vi "RangeCheck.vi"(0 "NhRegenGridSim in":refnum<class "NHRGridSim.lvclass">, 1 "RangeCheck":T1, 2 "Phase":i32, 3 "error in (no error)":errorcluster) -> (7 "NhRegenGridSim out":refnum<class "NHRGridSim.lvclass">, 10 "error out":errorcluster)   [LabVIEW 2018, in "AcPwrPlugins.lvlib" / "NHRGridSim.lvclass"]
doc: "This VI validates that the properties being set via the prefence dialog or stored in the INI file are valid."
uses:
  NHRGridSim.lvclass
  TypeDefs/RangeCheck.ctl
  <vilib>/Utility/error.llb/Error Cluster From Error Code.vi
  <vilib>/ErrorRing/Error Ring.xnode
  <instrlib>/NH Research 9400 Series/NH Research 9400 Series.lvlib
  <instrlib>/NH Research 9400 Series/Public/Utility/Query Capabilities (Frequency).vi
  <instrlib>/NH Research 9400 Series/Public/Utility/Query Capabilities (Power).vi
  <instrlib>/NH Research 9400 Series/Public/Utility/Query Capabilities (Current).vi
  <instrlib>/NH Research 9400 Series/Public/Utility/Query Capabilities (Voltage).vi
  <instrlib>/NH Research 9400 Series/Public/Utility/Query Capabilities (Phase Angle).vi
  <instrlib>/NH Research 9400 Series/Public/Utility/Query Capabilities (Sample).vi
  <instrlib>/NH Research 9400 Series/Public/Utility/Query Capabilities (Aperture).vi
  <instrlib>/NH Research 9400 Series/Public/Action-Status/Low Level/Query Range List (Voltage).vi
  <instrlib>/NH Research 9400 Series/Public/Action-Status/Low Level/Query Range List (Current).vi
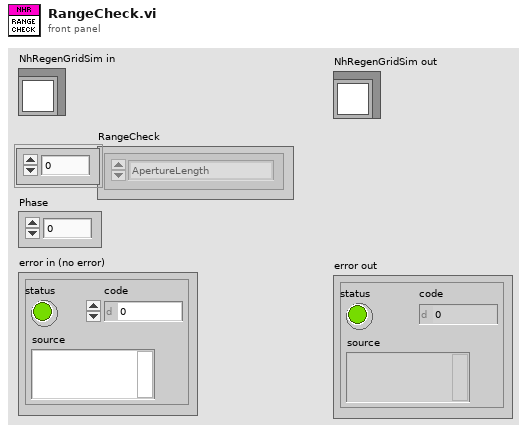
[diagram p1: front panel]
types:
  T1 = typedef "AcPwrPlugins.lvlib/NHRGridSim.lvclass/RangeCheck.ctl" = enum16{"ApertureLength", "NumberOfSamples", "SlewAngleMultiPhaseAB", "SlewAngleMultiPhaseAC", "RegulationGain", "VoltageRange", "CurrentRange", "PhaseAngle", "Power", "Current", "Voltage", "Frequency"}[]
  T2 = typedef "AcPwrPlugins.lvlib/NHRGridSim.lvclass/NHRGrid_Settings.ctl" = cluster{"MeasName":string, "Hardware":T3}
  T3 = typedef "AcPwrPlugins.lvlib/NHRGridSim.lvclass/NHRGrid_Hardware.ctl" = cluster{"Handle":string, "Reset":bool, "Mode":T4, "ID Query":bool, "Logical Instrument":T5}
  T4 = typedef "AcPwrPlugins.lvlib/NHRGridSim.lvclass/NHRGrid_Modes.ctl" = u8
  T5 = typedef "AcPwrPlugins.lvlib/NHRGridSim.lvclass/NHRGrid_Logical_Instrument.ctl" = cluster{"Name":string, "Vout (V)":dbl, "I limit (A)":dbl, "P limit (W)":dbl, "FreqOut (Hz)":dbl, "Ranges":cluster{"Voltage (V)":u16, "Current (A)":u16}, "Configure Instrument":u16, "Aperture (cycles)":i32, "AC Wave Shape":u16, "VType":string, "IType":string, "Phases":T6, "Slew Rates":T7, "Safety Trips":T8}[]
  T6 = typedef "AcPwrPlugins.lvlib/NHRGridSim.lvclass/NHRGrid_Phases.ctl" = cluster{"A-Volts (V)":dbl, "B-Volts (V)":dbl, "C-Volts (V)":dbl, "A-Curr (A)":dbl, "B-Curr (A)":dbl, "C-Curr (A)":dbl, "A-Power (W)":dbl, "B-Power (W)":dbl, "C-Power (W)":dbl, "Change at (Deg)":dbl, "B-Angle (Deg)":dbl, "C-Angle (Deg)":dbl}
  T7 = typedef "AcPwrPlugins.lvlib/NHRGridSim.lvclass/NHRGrid_SlewRates.ctl" = cluster{"Vmax (V/s)":dbl, "Vmin (V/s)":dbl, "Imax (A/s)":dbl, "Imin (A/s)":dbl, "Pmax (W/s)":dbl, "Pmin (W/s)":dbl, "Freq Max (Hz/s)":dbl, "Freq Min (Hz/s)":dbl, "Phase Angle Max (Deg/s)":dbl, "Phase Angle Min (Deg/s)":dbl}
  T8 = typedef "AcPwrPlugins.lvlib/NHRGridSim.lvclass/NHRGrid_SafetyTrips.ctl" = cluster{"Vmax (V)":dbl, "Vmin (V)":dbl, "Vmax Time (s)":dbl, "Vmin Time (s)":dbl, "Imax Source (A)":dbl, "Imax Sink (A)":dbl, "Imax Source Time (s)":dbl, "Imax Sink Time (s)":dbl, "Pmax Source (W)":dbl, "Pmax Sink (W)":dbl, "Pmax Source Time (s)":dbl, "Pmax Sink Time (s)":dbl, "Absolute Volt Peak":dbl, "Enable Volt Peak":bool, "Absolute Curr Peak":dbl, "Enable Curr Peak":bool}
  T9 = typedef "NH Research 9400 Series.lvlib/Range.ctl" = cluster{"Minimum":dbl, "Maximum":dbl}
  T10 = typedef "NH Research 9400 Series.lvlib/Current Capabilities.ctl" = cluster{"Module Min (A)":dbl, "Module Max (A)":dbl, "Range Min (A)":dbl, "Range Max (A)":dbl, "Measure Min (A)":dbl, "Measure Max (A)":dbl, "Measure Range Min (A)":dbl, "Measure Range Max (A)":dbl, "Slew Min (A per sec)":dbl, "Slew Max (A per sec)":dbl, "Slew Range Min (A per sec)":dbl, "Slew Range Max (A per sec)":dbl}
  T11 = typedef "NH Research 9400 Series.lvlib/Voltage Capabilities.ctl" = cluster{"Module Min (V)":dbl, "Module Max (V)":dbl, "Range Min (V)":dbl, "Range Max (V)":dbl, "Measure Min (V)":dbl, "Measure Max (V)":dbl, "Measure Range Min (V)":dbl, "Measure Range Max (V)":dbl, "Slew Min (V per sec)":dbl, "Slew Max (V per sec)":dbl, "Slew Range Min (V per sec)":dbl, "Slew Range Max (V per sec)":dbl}
  T12 = typedef "NH Research 9400 Series.lvlib/Power Capabilities.ctl" = cluster{"Module Min (W)":dbl, "Module Max (W)":dbl, "Range Min (W)":dbl, "Range Max (W)":dbl, "Slew Min (W per sec)":dbl, "Slew Max (W per sec)":dbl, "Slew Range Min (W per sec)":dbl, "Slew Range Max (W per sec)":dbl}
  T13 = typedef "NH Research 9400 Series.lvlib/Frequency Capabilities.ctl" = cluster{"Module Min (Hz)":dbl, "Module Max (Hz)":dbl, "Range Min (Hz)":dbl, "Range Max (Hz)":dbl, "Slew Min (Hz per sec)":dbl, "Slew Max (Hz per sec)":dbl, "Slew Range Min (Hz per sec)":dbl, "Slew Range Max (Hz per sec)":dbl}
  T14 = typedef "NH Research 9400 Series.lvlib/Phase Capabilities.ctl" = cluster{"Slew Min (deg per sec)":dbl, "Slew Max (deg per sec)":dbl, "Slew Range Min (deg per sec)":dbl, "Slew Range Max (deg per sec)":dbl}
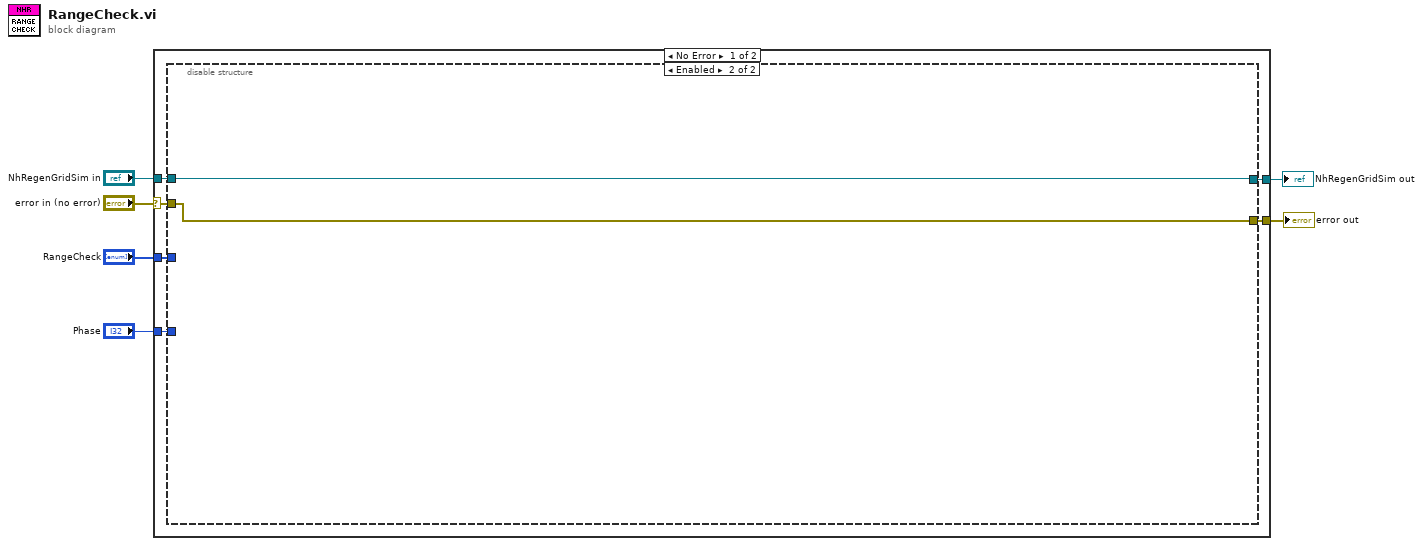
[diagram p0: block diagram]
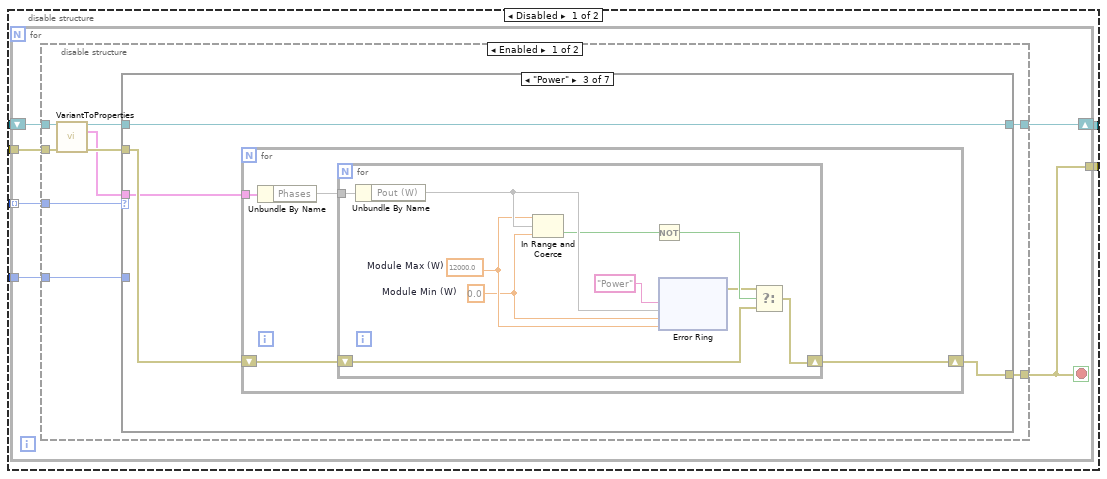
[diagram p2: hidden frame]
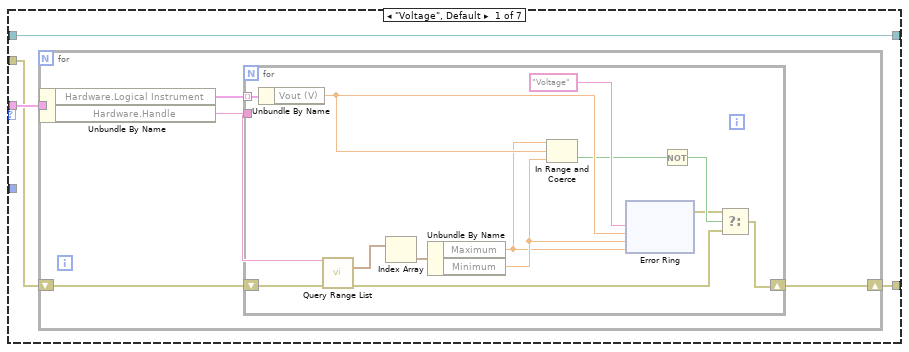
[diagram p3: hidden frame]
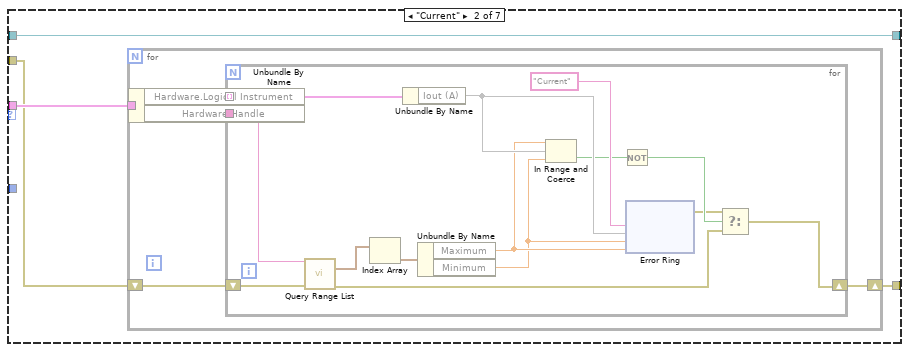
[diagram p4: hidden frame]
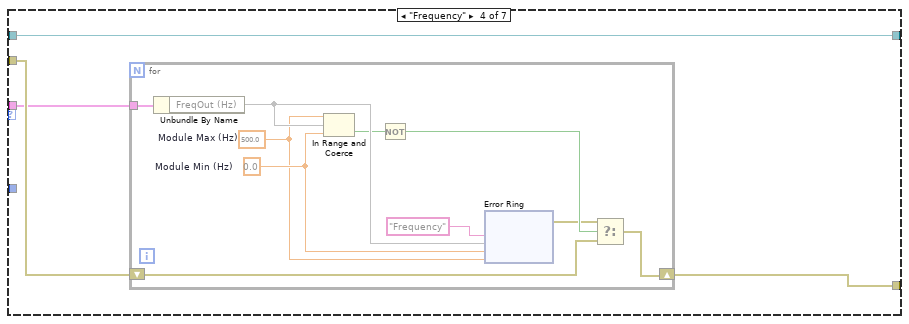
[diagram p5: hidden frame]
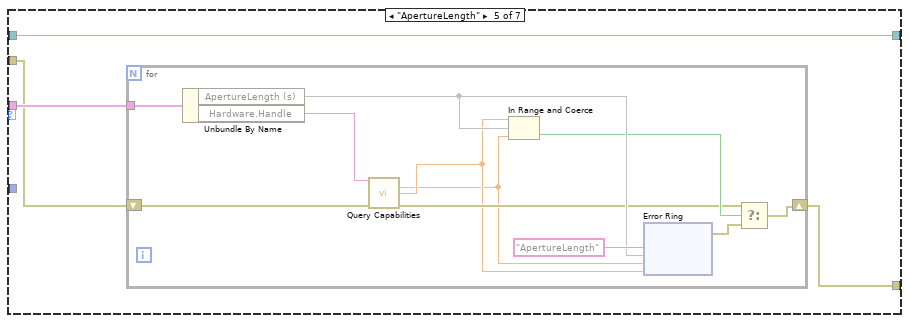
[diagram p6: hidden frame]
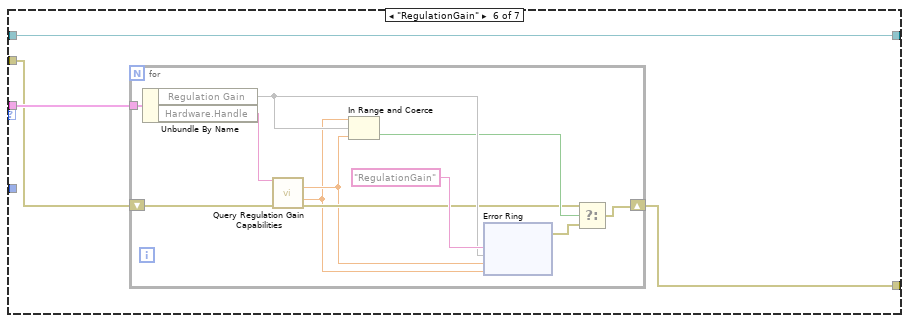
[diagram p7: hidden frame]
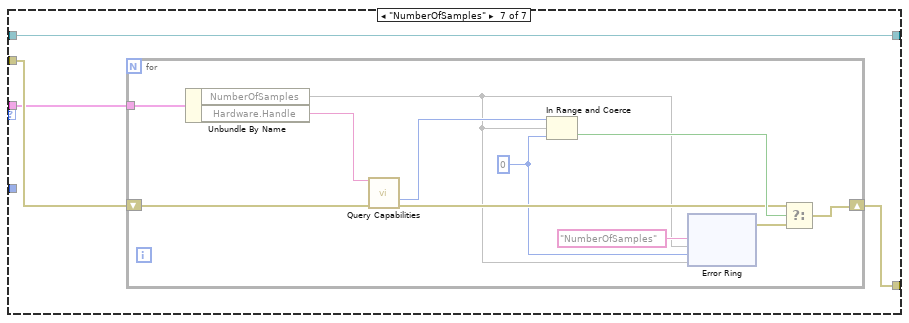
[diagram p8: hidden frame]
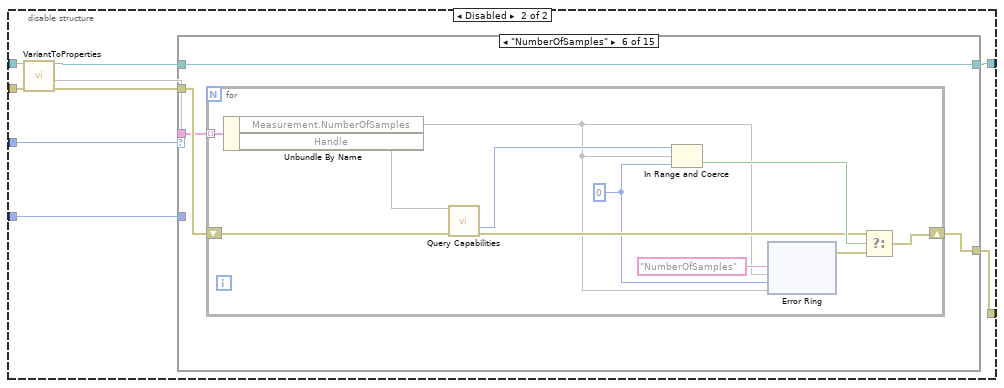
[diagram p9: hidden frame]
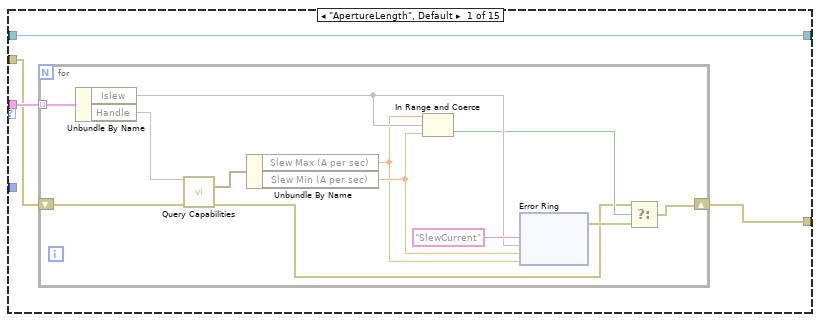
[diagram p10: hidden frame]
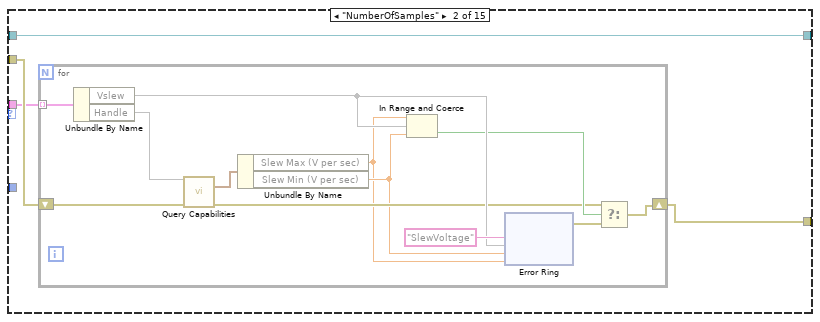
[diagram p11: hidden frame]
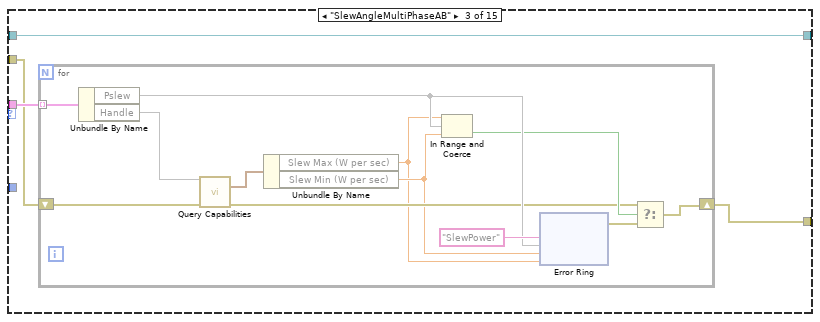
[diagram p12: hidden frame]
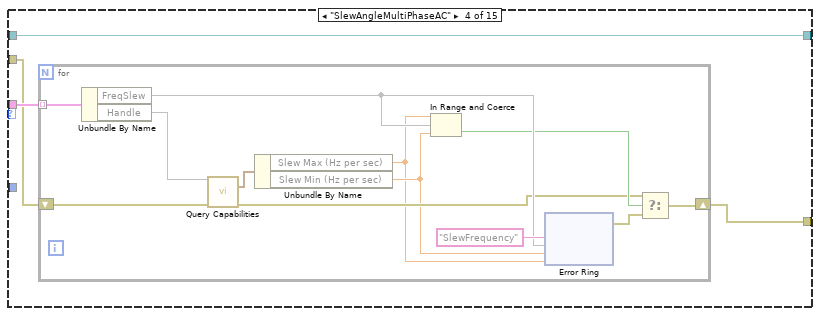
[diagram p13: hidden frame]
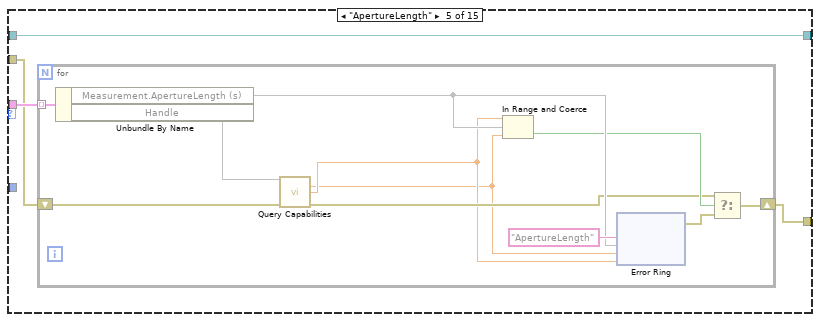
[diagram p14: hidden frame]
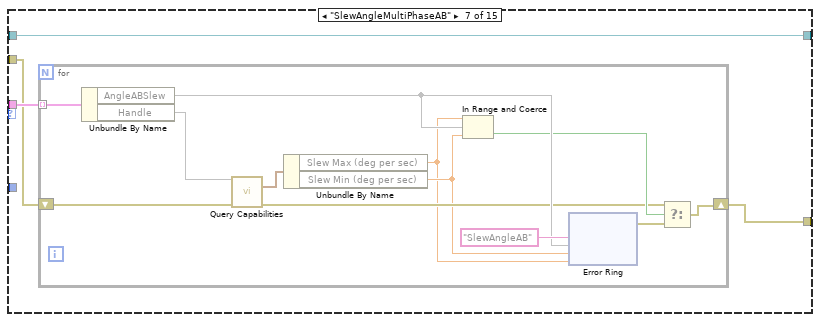
[diagram p15: hidden frame]
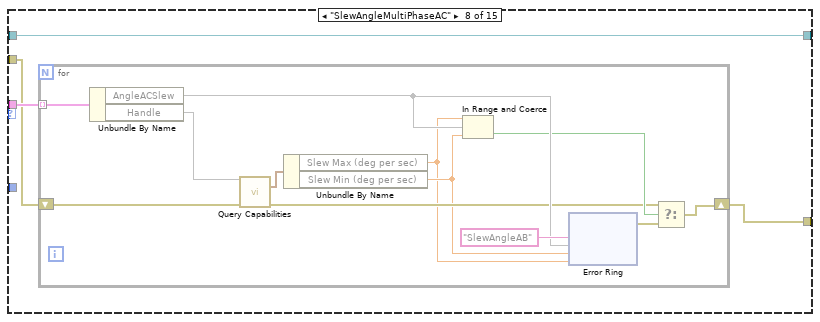
[diagram p16: hidden frame]
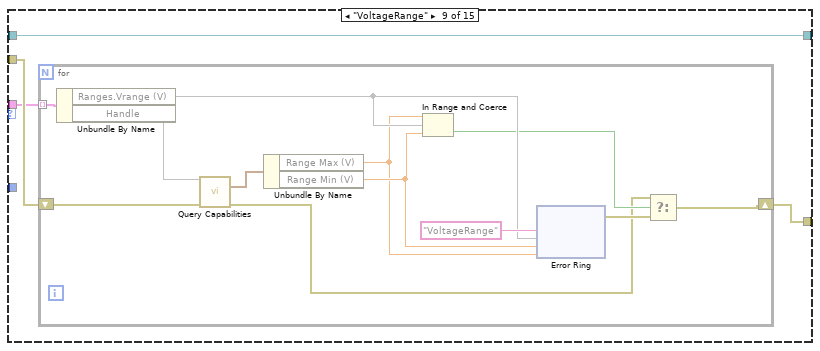
[diagram p17: hidden frame]
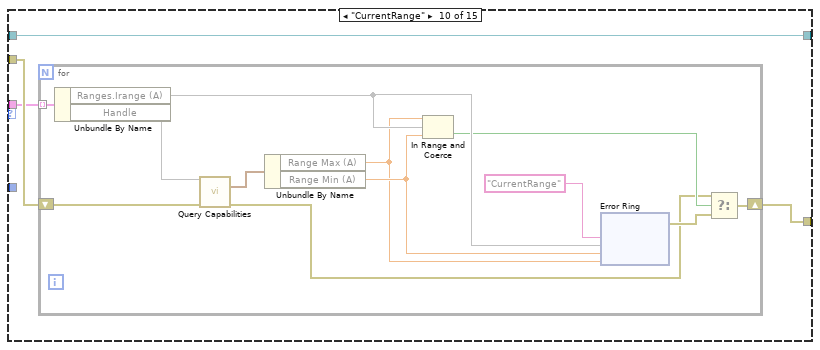
[diagram p18: hidden frame]
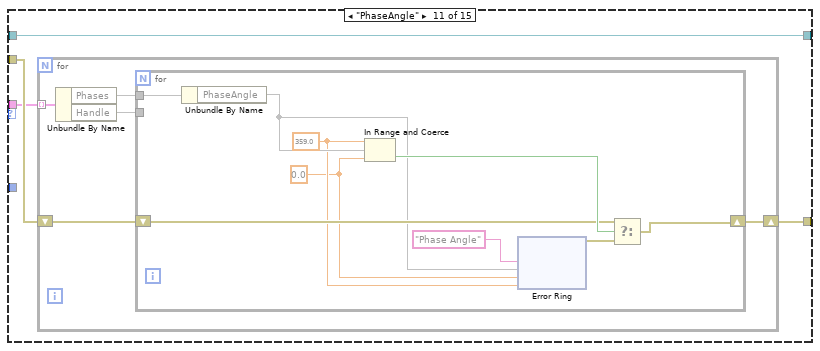
[diagram p19: hidden frame]
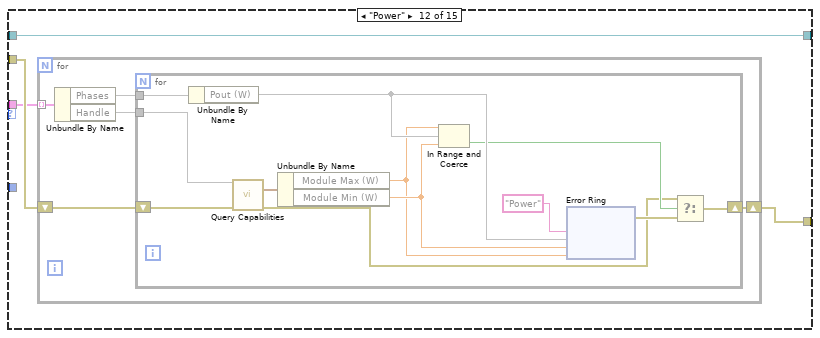
[diagram p20: hidden frame]
diagram:
  n1 = case shown="No Error" "error in (no error)" {
    selector: "error in (no error)" -> [w12 w641]
    tunnel: "Phase" -> [w11 _]
    tunnel: "NhRegenGridSim in" -> [w10 w642]
    tunnel: [w9 w642] -> w3
    tunnel: [w8 w641] -> w2
    tunnel: "RangeCheck" -> [w7 _]
    frame No Error {
      n2 = disable-structure shown="Enabled" {
        disable-tunnel: w12 -> [w18 w639]
        disable-tunnel: w11 -> [w17 _]
        disable-tunnel: w10 -> [w16 w640]
        disable-tunnel: [w15 w640] -> w9
        disable-tunnel: [w14 w639] -> w8
        disable-tunnel: w7 -> [w13 _]
        frame Disabled {
          n3 = for {
            tunnel: w13 -> [w24] mode=indexing
            tunnel: w17 -> [w23]
            shift-right: [w22] -> w15
            shift-left: w16 -> [w20]
            tunnel: [w21] -> w14
            tunnel: w18 -> [w19]
            stop <- w21 stop-if-true
            n4 = disable-structure shown="Enabled" {
              disable-tunnel: w24 -> [w33 w235]
              disable-tunnel: w23 -> [w32 w234]
              disable-tunnel: [w31 w233] -> w22
              disable-tunnel: [w30 w232] -> w21
              disable-tunnel: w20 -> [w29 w231]
              disable-tunnel: w19 -> [w28 w230]
              frame Enabled {
                n5 = call "VariantToProperties.vi"("NHRGridSim in"=w29, "error in (no error)"=w28) -> ("NHRGridSim out"=w26:refnum<class "NHRGridSim.lvclass">, "Device(s)Settings"=w25:T2, "error out"=w27:errorcluster)  [unwired: 8 in, 3 out]
                n6 = case shown="\"Power\"" w33 {
                  tunnel: w26 -> [w37 w70 w103 w130 w155 w180 w205]
                  tunnel: w32 -> [_ _ _ _ _ _ _]
                  tunnel: [w37 w70 w103 w130 w155 w180 w205] -> w31
                  tunnel: [w36 w69 w102 w131 w154 w179 w204] -> w30
                  tunnel: w27 -> [w34 w67 w101 w129 w152 w177 w203]
                  tunnel: w25 -> [w35 w68 w100 w128 w153 w178 w202]
                  frame "Voltage", Default {
                    n7 = for {
                      tunnel: w35 -> [w40]
                      shift-right: [w41] -> w36
                      shift-left: w34 -> [w42]
                      n8 = Unbundle By Name(w40) -> ("Hardware.Logical Instrument"=w39:T5, "Hardware.Handle"=w38:string)
                      n9 = for {
                        shift-right: [w55] -> w41
                        shift-left: w42 -> [w48]
                        tunnel: w39 -> [w54] mode=indexing
                        tunnel: w38 -> [w47]
                        n10 = Unbundle By Name(w54) -> ("Vout (V)"=w53:dbl)
                        n11 = call-poly <instrlib>:"Query Range List.vi"("VISA resource name"=w47, "error in (no error)"=w48) -> ("Voltage Range List (V)"=w46:T9[], "error out"=w49:errorcluster)  [unwired: 11 in, 1 out]
                        n12 = Index Array(array=w46) -> (element=w45:T9)  [unwired: 1 in]
                        n13 = Unbundle By Name(w45) -> ("Maximum"=w43:dbl, "Minimum"=w44:dbl)
                        n14 = In Range and Coerce(upper limit=w43, x=w53, lower limit=w44) -> (In Range?=w52:bool)  [unwired: 1 out]
                        n15 = xnode "Error Ring"("parameter 0"="Voltage", "parameter 1"=w53, "parameter 2"=w44, "parameter 3"=w43) -> ("error out"=w50:errorcluster)
                        n16 = Not(x=w52) -> (.not. x?=w51:bool)
                        n17 = Select(t=w50, s=w51, f=w49) -> (s? t:f=w55:errorcluster)
                      }
                    }
                  }
                  frame "Current" {
                    n18 = for {
                      tunnel: w68 -> [w73]
                      shift-right: [w74] -> w69
                      shift-left: w67 -> [w75]
                      n19 = Unbundle By Name(w73) -> ("Hardware.Logical Instrument"=w72:T5, "Hardware.Handle"=w71:string)
                      n20 = for {
                        shift-right: [w88] -> w74
                        shift-left: w75 -> [w81]
                        tunnel: w72 -> [w87] mode=indexing
                        tunnel: w71 -> [w79]
                        n21 = call-poly <instrlib>:"Query Range List.vi"("VISA resource name"=w79, "error in (no error)"=w81) -> ("Current Range List (A)"=w82:T9[], "error out"=w80:errorcluster)  [unwired: 11 in, 1 out]
                        n22 = Index Array(array=w82) -> (element=w78:T9)  [unwired: 1 in]
                        n23 = Unbundle By Name(w87) -> ("Iout (A)"=w86)
                        n24 = Unbundle By Name(w78) -> ("Maximum"=w77:dbl, "Minimum"=w76:dbl)
                        n25 = In Range and Coerce(upper limit=w77, x=w86, lower limit=w76) -> (In Range?=w85:bool)  [unwired: 1 out]
                        n26 = Not(x=w85) -> (.not. x?=w84:bool)
                        n27 = xnode "Error Ring"("parameter 0"="Current", "parameter 1"=w86, "parameter 2"=w76, "parameter 3"=w77) -> ("error out"=w83:errorcluster)
                        n28 = Select(t=w83, s=w84, f=w80) -> (s? t:f=w88:errorcluster)
                      }
                    }
                  }
                  frame "Power" {
                    n29 = for {
                      tunnel: w100 -> [w105]
                      shift-right: [w106] -> w102
                      shift-left: w101 -> [w107]
                      n30 = Unbundle By Name(w105) -> ("Phases"=w104)
                      n31 = for {
                        shift-right: [w116] -> w106
                        shift-left: w107 -> [w109]
                        tunnel: w104 -> [w115]
                        w112 = 0.0  # Module Min (W)
                        w113 = 12000.0  # Module Max (W)
                        n32 = Unbundle By Name(w115) -> ("Pout (W)"=w114)
                        n33 = In Range and Coerce(upper limit=w113, x=w114, lower limit=w112) -> (In Range?=w111:bool)  [unwired: 1 out]
                        n34 = Not(x=w111) -> (.not. x?=w110:bool)
                        n35 = xnode "Error Ring"("parameter 0"="Power", "parameter 1"=w114, "parameter 2"=w112, "parameter 3"=w113) -> ("error out"=w108:errorcluster)
                        n36 = Select(t=w108, s=w110, f=w109) -> (s? t:f=w116:errorcluster)
                      }
                    }
                  }
                  frame "Frequency" {
                    n37 = for {
                      tunnel: w128 -> [w139]
                      shift-right: [w140] -> w131
                      shift-left: w129 -> [w138]
                      w133 = 0.0  # Module Min (Hz)
                      w132 = 500.0  # Module Max (Hz)
                      n38 = Unbundle By Name(w139) -> ("FreqOut (Hz)"=w137)
                      n39 = In Range and Coerce(upper limit=w132, x=w137, lower limit=w133) -> (In Range?=w136:bool)  [unwired: 1 out]
                      n40 = Not(x=w136) -> (.not. x?=w135:bool)
                      n41 = xnode "Error Ring"("parameter 0"="Frequency", "parameter 1"=w137, "parameter 2"=w133, "parameter 3"=w132) -> ("error out"=w134:errorcluster)
                      n42 = Select(t=w134, s=w135, f=w138) -> (s? t:f=w140:errorcluster)
                    }
                  }
                  frame "ApertureLength" {
                    n43 = for {
                      tunnel: w153 -> [w163]
                      shift-right: [w164] -> w154
                      shift-left: w152 -> [w161]
                      n44 = Unbundle By Name(w163) -> ("ApertureLength (s)"=w160, "Hardware.Handle"=w162:string)
                      n45 = call-poly <instrlib>:"Query Capabilities.vi"("VISA resource name"=w162, "error in (no error)"=w161) -> ("Aperture Min (s)"=w156:dbl, "Aperture Max (s)"=w157:dbl, "error out"=w158:errorcluster)  [unwired: 10 in, 1 out]
                      n46 = In Range and Coerce(upper limit=w157, x=w160, lower limit=w156) -> (In Range?=w159:bool)  [unwired: 1 out]
                      n47 = xnode "Error Ring"("parameter 0"="ApertureLength", "parameter 1"=w160, "parameter 2"=w156, "parameter 3"=w157) -> ("error out"=w165:errorcluster)
                      n48 = Select(t=w158, s=w159, f=w165) -> (s? t:f=w164:errorcluster)
                    }
                  }
                  frame "RegulationGain" {
                    n49 = for {
                      tunnel: w178 -> [w188]
                      shift-right: [w189] -> w179
                      shift-left: w177 -> [w186]
                      n50 = Unbundle By Name(w188) -> ("Regulation Gain"=w185, "Hardware.Handle"=w187:string)
                      n51 = call <instrlib>:"Query Regulation Gain Capabilities.vi"("VISA resource name"=w187, "error in (no error)"=w186) -> ("Minimum"=w182:dbl, "Maximum"=w181:dbl, "error out"=w183:errorcluster)  [unwired: 9 in, 2 out]
                      n52 = In Range and Coerce(upper limit=w181, x=w185, lower limit=w182) -> (In Range?=w184:bool)  [unwired: 1 out]
                      n53 = xnode "Error Ring"("parameter 0"="RegulationGain", "parameter 1"=w185, "parameter 2"=w182, "parameter 3"=w181) -> ("error out"=w190:errorcluster)
                      n54 = Select(t=w183, s=w184, f=w190) -> (s? t:f=w189:errorcluster)
                    }
                  }
                  frame "NumberOfSamples" {
                    n55 = for {
                      tunnel: w202 -> [w213]
                      shift-right: [w214] -> w204
                      shift-left: w203 -> [w211]
                      w207 = u32 0 ("lower limit")
                      n56 = Unbundle By Name(w213) -> ("NumberOfSamples"=w206, "Hardware.Handle"=w212:string)
                      n57 = call-poly <instrlib>:"Query Capabilities.vi"("VISA resource name"=w212, "error in (no error)"=w211) -> ("Points"=w208:u32, "error out"=w209:errorcluster)  [unwired: 9 in, 3 out]
                      n58 = In Range and Coerce(upper limit=w208, x=w206, lower limit=w207) -> (In Range?=w210:bool)  [unwired: 1 out]
                      n59 = xnode "Error Ring"("parameter 0"="NumberOfSamples", "parameter 1"=w206, "parameter 2"=w207, "parameter 3"=w206) -> ("error out"=w215:errorcluster)
                      n60 = Select(t=w209, s=w210, f=w215) -> (s? t:f=w214:errorcluster)
                    }
                  }
                }
              }
              frame Disabled {
                n61 = call "VariantToProperties.vi"("NHRGridSim in"=w231, "error in (no error)"=w230) -> ("NHRGridSim out"=w228:refnum<class "NHRGridSim.lvclass">, 14:w227, "error out"=w229:errorcluster)  [unwired: 7 in, 4 out]
                n62 = case shown="\"NumberOfSamples\"" w235 {
                  tunnel: w228 -> [w239 w265 w291 w317 w343 w368 w393 w419 w445 w471 w497 w525 w556 w585 w615]
                  tunnel: w234 -> [_ _ _ _ _ _ _ _ _ _ _ _ _ _ _]
                  tunnel: [w239 w265 w291 w317 w343 w368 w393 w419 w445 w471 w497 w525 w556 w585 w615] -> w233
                  tunnel: [w238 w264 w290 w316 w342 w367 w392 w418 w444 w470 w496 w524 w555 w584 w616] -> w232
                  tunnel: w229 -> [w236 w263 w288 w314 w340 w366 w390 w416 w443 w469 w495 w523 w554 w582 w614]
                  tunnel: w227 -> [w237 w262 w289 w315 w341 w365 w391 w417 w442 w468 w494 w522 w553 w583 w613]
                  frame "ApertureLength", Default {
                    n63 = for {
                      tunnel: w237 -> [w248] mode=indexing
                      shift-right: [w249] -> w238
                      shift-left: w236 -> [w246]
                      n64 = Unbundle By Name(w248) -> ("Islew"=w244, "Handle"=w247)
                      n65 = call-poly <instrlib>:"Query Capabilities.vi"("VISA resource name"=w247, "error in (no error)"=w246) -> ("Current Capabilities"=w245:T10, "error out"=w240:errorcluster)  [unwired: 11 in, 1 out]
                      n66 = Unbundle By Name(w245) -> ("Slew Max (A per sec)"=w241:dbl, "Slew Min (A per sec)"=w242:dbl)
                      n67 = In Range and Coerce(upper limit=w241, x=w244, lower limit=w242) -> (In Range?=w243:bool)  [unwired: 1 out]
                      n68 = xnode "Error Ring"("parameter 0"="SlewCurrent", "parameter 1"=w244, "parameter 2"=w242, "parameter 3"=w241) -> ("error out"=w250:errorcluster)
                      n69 = Select(t=w240, s=w243, f=w250) -> (s? t:f=w249:errorcluster)
                    }
                  }
                  frame "NumberOfSamples" {
                    n70 = for {
                      tunnel: w262 -> [w274] mode=indexing
                      shift-right: [w275] -> w264
                      shift-left: w263 -> [w272]
                      n71 = Unbundle By Name(w274) -> ("Vslew"=w270, "Handle"=w273)
                      n72 = call-poly <instrlib>:"Query Capabilities.vi"("VISA resource name"=w273, "error in (no error)"=w272) -> ("Voltage Capabilities"=w271:T11, "error out"=w268:errorcluster)  [unwired: 11 in, 1 out]
                      n73 = Unbundle By Name(w271) -> ("Slew Max (V per sec)"=w266:dbl, "Slew Min (V per sec)"=w267:dbl)
                      n74 = In Range and Coerce(upper limit=w266, x=w270, lower limit=w267) -> (In Range?=w269:bool)  [unwired: 1 out]
                      n75 = xnode "Error Ring"("parameter 0"="SlewVoltage", "parameter 1"=w270, "parameter 2"=w267, "parameter 3"=w266) -> ("error out"=w276:errorcluster)
                      n76 = Select(t=w268, s=w269, f=w276) -> (s? t:f=w275:errorcluster)
                    }
                  }
                  frame "SlewAngleMultiPhaseAB" {
                    n77 = for {
                      tunnel: w289 -> [w300] mode=indexing
                      shift-right: [w301] -> w290
                      shift-left: w288 -> [w298]
                      n78 = Unbundle By Name(w300) -> ("Pslew"=w296, "Handle"=w299)
                      n79 = call-poly <instrlib>:"Query Capabilities.vi"("VISA resource name"=w299, "error in (no error)"=w298) -> ("Power Capabilities"=w297:T12, "error out"=w294:errorcluster)  [unwired: 11 in, 1 out]
                      n80 = Unbundle By Name(w297) -> ("Slew Max (W per sec)"=w292:dbl, "Slew Min (W per sec)"=w293:dbl)
                      n81 = In Range and Coerce(upper limit=w292, x=w296, lower limit=w293) -> (In Range?=w295:bool)  [unwired: 1 out]
                      n82 = xnode "Error Ring"("parameter 0"="SlewPower", "parameter 1"=w296, "parameter 2"=w293, "parameter 3"=w292) -> ("error out"=w302:errorcluster)
                      n83 = Select(t=w294, s=w295, f=w302) -> (s? t:f=w301:errorcluster)
                    }
                  }
                  frame "SlewAngleMultiPhaseAC" {
                    n84 = for {
                      tunnel: w315 -> [w326] mode=indexing
                      shift-right: [w327] -> w316
                      shift-left: w314 -> [w324]
                      n85 = Unbundle By Name(w326) -> ("FreqSlew"=w322, "Handle"=w325)
                      n86 = call-poly <instrlib>:"Query Capabilities.vi"("VISA resource name"=w325, "error in (no error)"=w324) -> ("Frequency Capabilities"=w323:T13, "error out"=w320:errorcluster)  [unwired: 11 in, 1 out]
                      n87 = Unbundle By Name(w323) -> ("Slew Max (Hz per sec)"=w318:dbl, "Slew Min (Hz per sec)"=w319:dbl)
                      n88 = In Range and Coerce(upper limit=w318, x=w322, lower limit=w319) -> (In Range?=w321:bool)  [unwired: 1 out]
                      n89 = xnode "Error Ring"("parameter 0"="SlewFrequency", "parameter 1"=w322, "parameter 2"=w319, "parameter 3"=w318) -> ("error out"=w328:errorcluster)
                      n90 = Select(t=w320, s=w321, f=w328) -> (s? t:f=w327:errorcluster)
                    }
                  }
                  frame "ApertureLength" {
                    n91 = for {
                      tunnel: w341 -> [w351] mode=indexing
                      shift-right: [w352] -> w342
                      shift-left: w340 -> [w349]
                      n92 = Unbundle By Name(w351) -> ("Measurement.ApertureLength (s)"=w348, "Handle"=w350)
                      n93 = call-poly <instrlib>:"Query Capabilities.vi"("VISA resource name"=w350, "error in (no error)"=w349) -> ("Aperture Min (s)"=w344:dbl, "Aperture Max (s)"=w345:dbl, "error out"=w346:errorcluster)  [unwired: 10 in, 1 out]
                      n94 = In Range and Coerce(upper limit=w345, x=w348, lower limit=w344) -> (In Range?=w347:bool)  [unwired: 1 out]
                      n95 = xnode "Error Ring"("parameter 0"="ApertureLength", "parameter 1"=w348, "parameter 2"=w344, "parameter 3"=w345) -> ("error out"=w353:errorcluster)
                      n96 = Select(t=w346, s=w347, f=w353) -> (s? t:f=w352:errorcluster)
                    }
                  }
                  frame "NumberOfSamples" {
                    n97 = for {
                      tunnel: w365 -> [w376] mode=indexing
                      shift-right: [w377] -> w367
                      shift-left: w366 -> [w374]
                      w370 = u32 0 ("lower limit")
                      n98 = Unbundle By Name(w376) -> ("Measurement.NumberOfSamples"=w369, "Handle"=w375)
                      n99 = call-poly <instrlib>:"Query Capabilities.vi"("VISA resource name"=w375, "error in (no error)"=w374) -> ("Points"=w371:u32, "error out"=w372:errorcluster)  [unwired: 9 in, 3 out]
                      n100 = In Range and Coerce(upper limit=w371, x=w369, lower limit=w370) -> (In Range?=w373:bool)  [unwired: 1 out]
                      n101 = xnode "Error Ring"("parameter 0"="NumberOfSamples", "parameter 1"=w369, "parameter 2"=w370, "parameter 3"=w369) -> ("error out"=w378:errorcluster)
                      n102 = Select(t=w372, s=w373, f=w378) -> (s? t:f=w377:errorcluster)
                    }
                  }
                  frame "SlewAngleMultiPhaseAB" {
                    n103 = for {
                      tunnel: w391 -> [w402] mode=indexing
                      shift-right: [w403] -> w392
                      shift-left: w390 -> [w400]
                      n104 = Unbundle By Name(w402) -> ("AngleABSlew"=w398, "Handle"=w401)
                      n105 = call-poly <instrlib>:"Query Capabilities.vi"("VISA resource name"=w401, "error in (no error)"=w400) -> ("Phase Angle Capabilities"=w399:T14, "error out"=w396:errorcluster)  [unwired: 11 in, 1 out]
                      n106 = Unbundle By Name(w399) -> ("Slew Max (deg per sec)"=w394:dbl, "Slew Min (deg per sec)"=w395:dbl)
                      n107 = In Range and Coerce(upper limit=w394, x=w398, lower limit=w395) -> (In Range?=w397:bool)  [unwired: 1 out]
                      n108 = xnode "Error Ring"("parameter 0"="SlewAngleAB", "parameter 1"=w398, "parameter 2"=w395, "parameter 3"=w394) -> ("error out"=w404:errorcluster)
                      n109 = Select(t=w396, s=w397, f=w404) -> (s? t:f=w403:errorcluster)
                    }
                  }
                  frame "SlewAngleMultiPhaseAC" {
                    n110 = for {
                      tunnel: w417 -> [w428] mode=indexing
                      shift-right: [w429] -> w418
                      shift-left: w416 -> [w426]
                      n111 = Unbundle By Name(w428) -> ("AngleACSlew"=w424, "Handle"=w427)
                      n112 = call-poly <instrlib>:"Query Capabilities.vi"("VISA resource name"=w427, "error in (no error)"=w426) -> ("Phase Angle Capabilities"=w425:T14, "error out"=w422:errorcluster)  [unwired: 11 in, 1 out]
                      n113 = Unbundle By Name(w425) -> ("Slew Max (deg per sec)"=w420:dbl, "Slew Min (deg per sec)"=w421:dbl)
                      n114 = In Range and Coerce(upper limit=w420, x=w424, lower limit=w421) -> (In Range?=w423:bool)  [unwired: 1 out]
                      n115 = xnode "Error Ring"("parameter 0"="SlewAngleAB", "parameter 1"=w424, "parameter 2"=w421, "parameter 3"=w420) -> ("error out"=w430:errorcluster)
                      n116 = Select(t=w422, s=w423, f=w430) -> (s? t:f=w429:errorcluster)
                    }
                  }
                  frame "VoltageRange" {
                    n117 = for {
                      tunnel: w442 -> [w454] mode=indexing
                      shift-right: [w455] -> w444
                      shift-left: w443 -> [w452]
                      n118 = Unbundle By Name(w454) -> ("Ranges.Vrange (V)"=w450, "Handle"=w453)
                      n119 = call-poly <instrlib>:"Query Capabilities.vi"("VISA resource name"=w453, "error in (no error)"=w452) -> ("Voltage Capabilities"=w451:T11, "error out"=w446:errorcluster)  [unwired: 11 in, 1 out]
                      n120 = Unbundle By Name(w451) -> ("Range Max (V)"=w447:dbl, "Range Min (V)"=w448:dbl)
                      n121 = In Range and Coerce(upper limit=w447, x=w450, lower limit=w448) -> (In Range?=w449:bool)  [unwired: 1 out]
                      n122 = xnode "Error Ring"("parameter 0"="VoltageRange", "parameter 1"=w450, "parameter 2"=w448, "parameter 3"=w447) -> ("error out"=w456:errorcluster)
                      n123 = Select(t=w446, s=w449, f=w456) -> (s? t:f=w455:errorcluster)
                    }
                  }
                  frame "CurrentRange" {
                    n124 = for {
                      tunnel: w468 -> [w480] mode=indexing
                      shift-right: [w481] -> w470
                      shift-left: w469 -> [w478]
                      n125 = Unbundle By Name(w480) -> ("Ranges.Irange (A)"=w476, "Handle"=w479)
                      n126 = call-poly <instrlib>:"Query Capabilities.vi"("VISA resource name"=w479, "error in (no error)"=w478) -> ("Current Capabilities"=w477:T10, "error out"=w472:errorcluster)  [unwired: 11 in, 1 out]
                      n127 = Unbundle By Name(w477) -> ("Range Max (A)"=w473:dbl, "Range Min (A)"=w474:dbl)
                      n128 = In Range and Coerce(upper limit=w473, x=w476, lower limit=w474) -> (In Range?=w475:bool)  [unwired: 1 out]
                      n129 = xnode "Error Ring"("parameter 0"="CurrentRange", "parameter 1"=w476, "parameter 2"=w474, "parameter 3"=w473) -> ("error out"=w482:errorcluster)
                      n130 = Select(t=w472, s=w475, f=w482) -> (s? t:f=w481:errorcluster)
                    }
                  }
                  frame "PhaseAngle" {
                    n131 = for {
                      tunnel: w494 -> [w500] mode=indexing
                      shift-right: [w501] -> w496
                      shift-left: w495 -> [w502]
                      n132 = Unbundle By Name(w500) -> ("Phases"=w499, "Handle"=w498)
                      n133 = for {
                        shift-right: [w509] -> w501
                        shift-left: w502 -> [w506]
                        tunnel: w499 -> [w508]
                        tunnel: w498 -> [_]
                        w504 = 359.0 ("Slew Max (deg per sec)")
                        w503 = 0.0 ("Slew Max (deg per sec)")
                        n134 = Unbundle By Name(w508) -> ("PhaseAngle"=w505)
                        n135 = In Range and Coerce(upper limit=w504, x=w505, lower limit=w503) -> (In Range?=w507:bool)  [unwired: 1 out]
                        n136 = xnode "Error Ring"("parameter 0"="Phase Angle", "parameter 1"=w505, "parameter 2"=w503, "parameter 3"=w504) -> ("error out"=w510:errorcluster)
                        n137 = Select(t=w506, s=w507, f=w510) -> (s? t:f=w509:errorcluster)
                      }
                    }
                  }
                  frame "Power" {
                    n138 = for {
                      tunnel: w522 -> [w528] mode=indexing
                      shift-right: [w529] -> w524
                      shift-left: w523 -> [w530]
                      n139 = Unbundle By Name(w528) -> ("Phases"=w527, "Handle"=w526)
                      n140 = for {
                        shift-right: [w540] -> w529
                        shift-left: w530 -> [w535]
                        tunnel: w527 -> [w539]
                        tunnel: w526 -> [w534]
                        n141 = Unbundle By Name(w539) -> ("Pout (W)"=w538)
                        n142 = call-poly <instrlib>:"Query Capabilities.vi"("VISA resource name"=w534, "error in (no error)"=w535) -> ("Power Capabilities"=w536:T12, "error out"=w533:errorcluster)  [unwired: 11 in, 1 out]
                        n143 = Unbundle By Name(w536) -> ("Module Max (W)"=w531:dbl, "Module Min (W)"=w532:dbl)
                        n144 = In Range and Coerce(upper limit=w531, x=w538, lower limit=w532) -> (In Range?=w537:bool)  [unwired: 1 out]
                        n145 = xnode "Error Ring"("parameter 0"="Power", "parameter 1"=w538, "parameter 2"=w532, "parameter 3"=w531) -> ("error out"=w541:errorcluster)
                        n146 = Select(t=w533, s=w537, f=w541) -> (s? t:f=w540:errorcluster)
                      }
                    }
                  }
                  frame "Current" {
                    n147 = for {
                      tunnel: w553 -> [w559] mode=indexing
                      shift-right: [w560] -> w555
                      shift-left: w554 -> [w561]
                      n148 = Unbundle By Name(w559) -> ("Phases"=w558, "Handle"=w557)
                      n149 = for {
                        shift-right: [w571] -> w560
                        shift-left: w561 -> [w566]
                        tunnel: w558 -> [w570]
                        tunnel: w557 -> [w565]
                        n150 = Unbundle By Name(w570) -> ("Iout (A)"=w569)
                        n151 = call-poly <instrlib>:"Query Capabilities.vi"("VISA resource name"=w565, "error in (no error)"=w566) -> ("Current Capabilities"=w567:T10, "error out"=w564:errorcluster)  [unwired: 11 in, 1 out]
                        n152 = Unbundle By Name(w567) -> ("Module Max (A)"=w562:dbl, "Module Min (A)"=w563:dbl)
                        n153 = In Range and Coerce(upper limit=w562, x=w569, lower limit=w563) -> (In Range?=w568:bool)  [unwired: 1 out]
                        n154 = xnode "Error Ring"("parameter 0"="Current", "parameter 1"=w569, "parameter 2"=w563, "parameter 3"=w562) -> ("error out"=w572:errorcluster)
                        n155 = Select(t=w564, s=w568, f=w572) -> (s? t:f=w571:errorcluster)
                      }
                    }
                  }
                  frame "Voltage" {
                    n156 = for {
                      tunnel: w583 -> [w588] mode=indexing
                      shift-right: [w589] -> w584
                      shift-left: w582 -> [w590]
                      n157 = Unbundle By Name(w588) -> ("Phases"=w587, "Handle"=w586)
                      n158 = for {
                        shift-right: [w600] -> w589
                        shift-left: w590 -> [w595]
                        tunnel: w587 -> [w599]
                        tunnel: w586 -> [w594]
                        n159 = Unbundle By Name(w599) -> ("Vout (V)"=w598)
                        n160 = call-poly <instrlib>:"Query Capabilities.vi"("VISA resource name"=w594, "error in (no error)"=w595) -> ("Voltage Capabilities"=w596:T11, "error out"=w593:errorcluster)  [unwired: 11 in, 1 out]
                        n161 = Unbundle By Name(w596) -> ("Module Max (V)"=w592:dbl, "Module Min (V)"=w591:dbl)
                        n162 = In Range and Coerce(upper limit=w592, x=w598, lower limit=w591) -> (In Range?=w597:bool)  [unwired: 1 out]
                        n163 = xnode "Error Ring"("parameter 0"="Voltage", "parameter 1"=w598, "parameter 2"=w591, "parameter 3"=w592) -> ("error out"=w601:errorcluster)
                        n164 = Select(t=w593, s=w597, f=w601) -> (s? t:f=w600:errorcluster)
                      }
                    }
                  }
                  frame "Frequency" {
                    n165 = for {
                      tunnel: w613 -> [w625] mode=indexing
                      shift-right: [w626] -> w616
                      shift-left: w614 -> [w623]
                      n166 = Unbundle By Name(w625) -> ("FreqOut (Hz)"=w621, "Handle"=w624)
                      n167 = call-poly <instrlib>:"Query Capabilities.vi"("VISA resource name"=w624, "error in (no error)"=w623) -> ("Frequency Capabilities"=w622:T13, "error out"=w617:errorcluster)  [unwired: 11 in, 1 out]
                      n168 = Unbundle By Name(w622) -> ("Module Max (Hz)"=w618:dbl, "Module Min (Hz)"=w619:dbl)
                      n169 = In Range and Coerce(upper limit=w618, x=w621, lower limit=w619) -> (In Range?=w620:bool)  [unwired: 1 out]
                      n170 = xnode "Error Ring"("parameter 0"="Frequency", "parameter 1"=w621, "parameter 2"=w619, "parameter 3"=w618) -> ("error out"=w627:errorcluster)
                      n171 = Select(t=w617, s=w620, f=w627) -> (s? t:f=w626:errorcluster)
                    }
                  }
                }
              }
            }
          }
        }
        frame Enabled {
        }
      }
    }
    frame Error {
    }
  }
  "NhRegenGridSim out" <- w3
  "error out" <- w2
